vi "Fetch Multi Eval Meas List EVM RMS Results.vi"(6 "Window Position (Low)":i32(ring) items=["Low", "High"], 8 "error in (no error)":errorcluster, 9 "Result Type (Current)":i32(ring) items=["Current", "Average", "Extreme", "Standard Deviation"], 10 "Instance (1)":T1=1, 11 "VISA resource name":refnum<visa-resource-name>) -> (0 "error out":errorcluster, 1 "Results":dbl[](array[numeric]) format="%^.3e", 2 "Reliability":i32, 3 "VISA resource name out":refnum<visa-resource-name>)   [LabVIEW 2020, in "Rohde&Schwarz CMWXP NR FR1 Measurement.lvlib"]
doc: "Return error vector magnitude RMS values for low and high EVM window position, for all measured list mode segments.\n\nAttributes:\nRSCMWXPNRFR1M_ATTR_FETCH_MULTI_EVAL_MEAS_LIST_EVM_RMS_LOW_CURRENT_RESULTS\nRSCMWXPNRFR1M_ATTR_FETCH_MULTI_EVAL_MEAS_LIST_EVM_RMS_LOW_AVERAGE_RESULTS\nRSCMWXPNRFR1M_ATTR_FETCH_MULTI_EVAL_MEAS_LIST_EVM_RMS_LOW_EXTREME_RESULTS\nRSCMWXPNRFR1M_ATTR_FETCH_MULTI_EVAL_MEAS_LIST_EVM_RMS_LOW_STANDARD_DEVIATION_RESULTS\nRSCMWXPNRFR1M_ATTR_FETCH_MULTI_EVAL_MEAS_LIST_EVM_RMS_HIGH_CURRENT_RESULTS\nRSCMWXPNRFR1M_ATTR_FETCH_MULTI_EVAL_MEAS_LIST_EVM_RMS_HIGH_AVERAGE_RESULTS\nRSCMWXPNRFR1M_ATTR_FETCH_MULTI_EVAL_MEAS_LIST_EVM_RMS_HIGH_EXTREME_RESULTS\nRSCMWXPNRFR1M_ATTR_FETCH_MULTI_EVAL_MEAS_LIST_EVM_RMS_HIGH_STANDARD_DEVIATION_RESULTS\n\nRemote-control commands:\nFETCh:NRSub:MEAS<i>:MEValuation:LIST:MODulation:EVM:RMS:LOW:CURRent?\nFETCh:NRSub:MEAS<i>:MEValuation:LIST:MODulation:EVM:RMS:LOW:AVERage?\nFETCh:NRSub:MEAS<i>:MEValuation:LIST:MODulation:EVM:RMS:LOW:EXTReme?\nFETCh:NRSub:MEAS<i>:MEValuation:LIST:MODulation:EVM:RMS:LOW:SDEViation?\nFETCh:NRSub:MEAS<i>:MEValuation:LIST:MODulation:EVM:RMS:HIGH:CURRent?\nFETCh:NRSub:MEAS<i>:MEValuation:LIST:MODulation:EVM:RMS:HIGH:AVERage?\nFETCh:NRSub:MEAS<i>:MEValuation:LIST:MODulation:EVM:RMS:HIGH:EXTReme?\nFETCh:NRSub:MEAS<i>:MEValuation:LIST:MODulation:EVM:RMS:HIGH:SDEViation?"
uses:
  <instrlib>/Rohde&Schwarz CMWXP NR FR1 Measurement/Rohde&Schwarz CMWXP NR FR1 Measurement.lvlib
  <instrlib>/Rohde&Schwarz CMWXP NR FR1 Measurement/Private/_Instance.ctl
  <instrlib>/Rohde&Schwarz CMWXP NR FR1 Measurement/Private/rsidr_core.llb/rsidr_core.lvlib
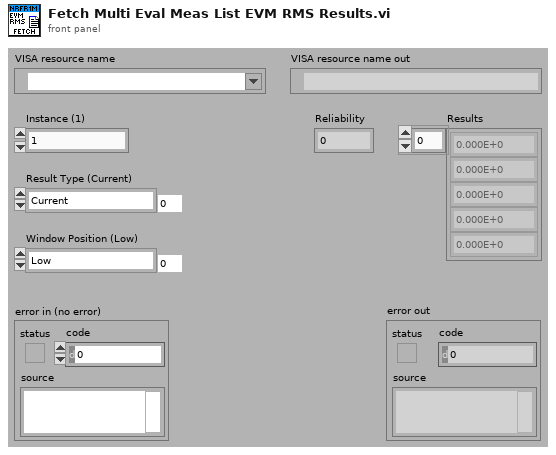
[diagram p1: front panel]
types:
  T1 = typedef "Rohde&Schwarz CMWXP NR FR1 Measurement.lvlib/_Instance.ctl" = i32
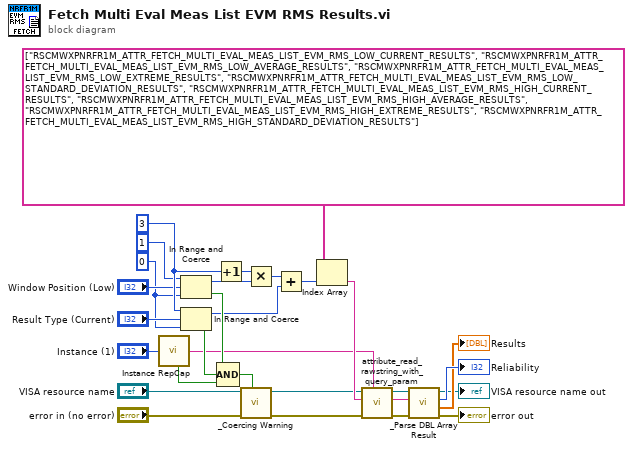
[diagram p0: block diagram]
diagram:
  w21 = 3
  w19 = 0
  n1 = call <instrlib>:"Instance RepCap.vi"("Instance In"="Instance (1)") -> ("In Range?"=w24:bool, "RepCap Identifier Out"=w8:string)  [unwired: 1 in]
  n2 = In Range and Coerce(upper limit=1, x="Window Position (Low)", lower limit=w19) -> (coerced(x)=w15:i32, In Range?=w16:bool)
  n3 = In Range and Coerce(upper limit=w21, x="Result Type (Current)", lower limit=w19) -> (coerced(x)=w14:i32, In Range?=w17:bool)
  n4 = Increment(x=w21) -> (x+1=w22:i32)
  n5 = Compound Arithmetic op=AND(w16, w17, w24) -> (w25:bool)
  n6 = call <instrlib>:"_Coercing Warning.vi"("In Range?"=w25, "error in (no error)"="error in (no error)", "VISA resource name"="VISA resource name") -> ("error out"=w9:errorcluster, "VISA resource name out"=w10:refnum<visa-resource-name>)  [unwired: 7 in]
  n7 = Multiply(x=w22, y=w15) -> (x*y=w26:i32)
  n8 = Add(x=w26, y=w14) -> (x+y=w13:i32)
  n9 = Index Array(array=string[] ["RSCMWXPNRFR1M_ATTR_FETCH_MULTI_EVAL_MEAS_LIST_EVM_RMS_LOW_CURRENT_RESULTS", "RSCMWXPNRFR1M_ATTR_FETCH_MULTI_EVAL_MEAS_LIST_EVM_RMS_LOW_AVERAGE_RESULTS", "RSCMWXPNRFR1M_ATTR_FETCH_MULTI_EVAL_MEAS_LIST_EVM_RMS_LOW_EXTREME_RESULTS", "RSCMWXPNRFR1M_ATTR_FETCH_MULTI_EVAL_MEAS_LIST_EVM_RMS_LOW_STANDARD_DEVIATION_RESULTS", "RSCMWXPNRFR1M_ATTR_FETCH_MULTI_EVAL_MEAS_LIST_EVM_RMS_HIGH_CURRENT_RESULTS", "RSCMWXPNRFR1M_ATTR_FETCH_MULTI_EVAL_MEAS_LIST_EVM_RMS_HIGH_AVERAGE_RESULTS", "RSCMWXPNRFR1M_ATTR_FETCH_MULTI_EVAL_MEAS_LIST_EVM_RMS_HIGH_EXTREME_RESULTS", "RSCMWXPNRFR1M_ATTR_FETCH_MULTI_EVAL_MEAS_LIST_EVM_RMS_HIGH_STANDARD_DEVIATION_RESULTS"], index=w13) -> (element=w11:string)
  n10 = call <instrlib>:"attribute_read_rawstring_with_query_param.vi"("Repeated Capability"=w8, "error in"=w9, "Attribute ID"=w11, "VISA resource name"=w10) -> ("error out"=w7:errorcluster, "Raw String out"=w6:string, "VISA resource name out"=w5:refnum<visa-resource-name>)  [unwired: 5 in]
  n11 = call <instrlib>:"_Parse DBL Array Result.vi"("error in (no error)"=w7, "Input String"=w6, "VISA resource name"=w5) -> ("error out"=→"error out":errorcluster, "Results"=→"Results":dbl[], "Reliability"=→"Reliability":i32, "VISA resource name out"=→"VISA resource name out":refnum<visa-resource-name>)  [unwired: 5 in]
